vi "Write Analog Data.vi"(8 "error in (no error)":errorcluster, 10 "Analog Data":waveform(dbl)[](array[waveform]), 11 "Analog Input Waveform Data Msg in":refnum<class "Analog Input Waveform Data Msg.lvclass">) -> (0 "error out":errorcluster, 3 "Analog Input Waveform Data Msg out":refnum<class "Analog Input Waveform Data Msg.lvclass">)   [LabVIEW 2024, in "DAQmx Actor Interface.lvlib" / "Analog Input Waveform Data Msg.lvclass"]
uses:
  Analog Input Waveform Data Msg.lvclass
  Analog Input Waveform Data Msg.lvclass/Analog Input Waveform Data Msg.ctl
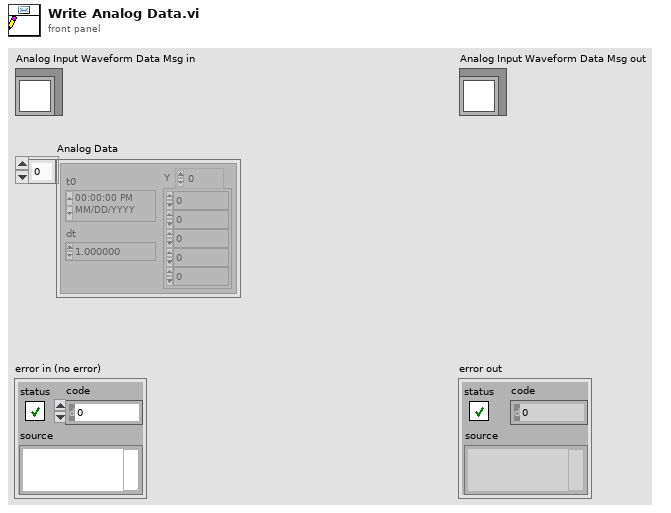
[diagram p1: front panel]
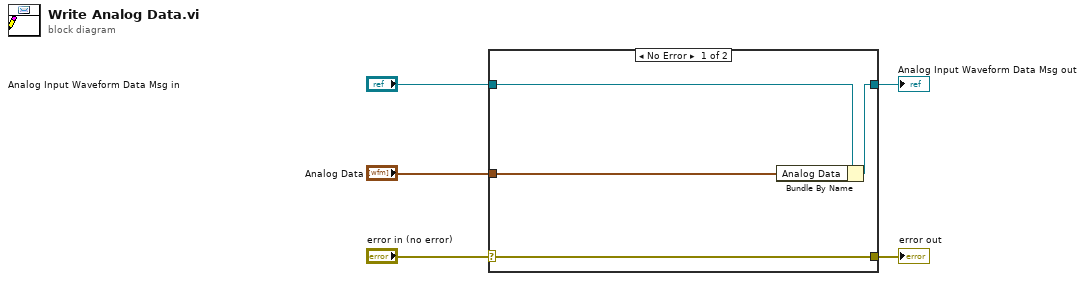
[diagram p0: block diagram]
diagram:
  n1 = case shown="No Error" "error in (no error)" {
    selector: "error in (no error)" -> [w9 w10]
    tunnel: [w9 w10] -> w4
    tunnel: [w7 w11] -> w2
    tunnel: "Analog Input Waveform Data Msg in" -> [w8 w11]
    tunnel: "Analog Data" -> [w6 _]
    frame No Error {
      n2 = Bundle By Name(cluster=w8, "Analog Data"=w6) -> (w7:refnum<class "Analog Input Waveform Data Msg.lvclass">)
    }
    frame Error {
    }
  }
  "error out" <- w4
  "Analog Input Waveform Data Msg out" <- w2
